vi "Split Single-line Message.vi"(2 "single-line text":string) -> (6 "operator":string, 7 "state":string, 9 "args":string, 10 "source/target":string)   [LabVIEW 2017, in "CSM Shared.lvlib"]
uses:
  CSM Shared.lvlib
  <vilib>/regexp/Match Regular Expression.xnode
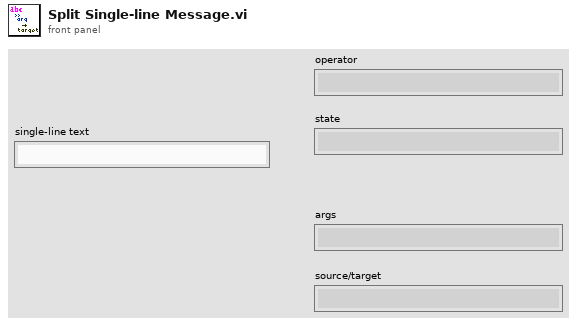
[diagram p1: front panel]
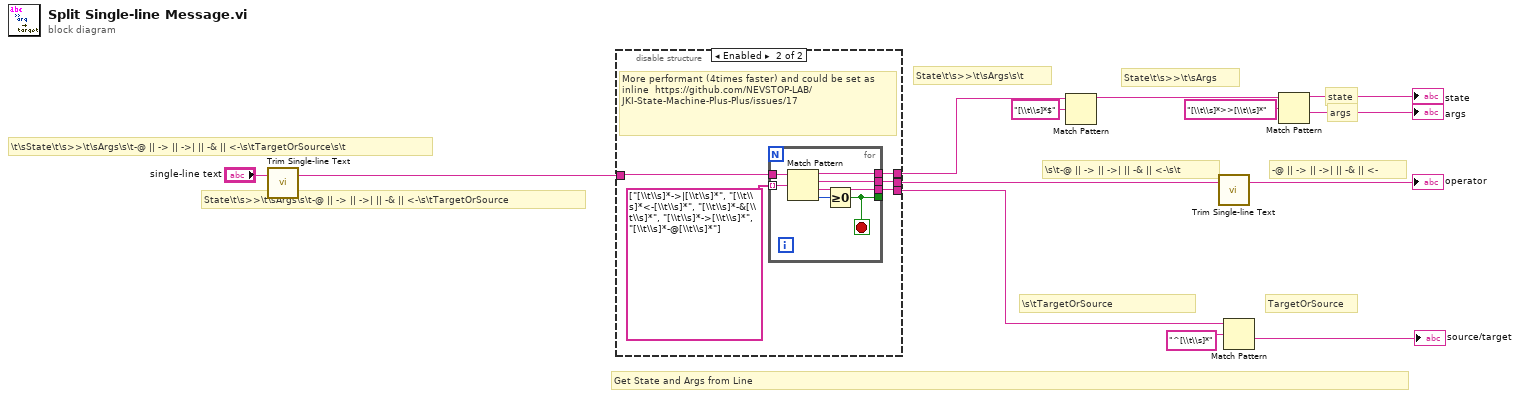
[diagram p0: block diagram]
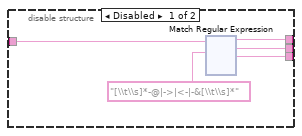
[diagram p2: hidden frame]
diagram:
  # "TargetOrSource"
  # "\\t\\sState\\t\\s>>\\t\\sArgs\\s\\t-@ || -> || ->| || -& || <-\\s\\tTargetOrSource\\s\\t"
  # "-@ || -> || ->| || -& || <-"
  # "\\s\\t-@ || -> || ->| || -& || <-\\s\\t"
  # "State\\t\\s>>\\t\\sArgs"
  # "State\\t\\s>>\\t\\sArgs\\s\\t"
  # "Get State and Args from Line"
  # "State\\t\\s>>\\t\\sArgs\\s\\t-@ || -> || ->| || -& || <-\\s\\tTargetOrSource"
  # "\\s\\tTargetOrSource"
  # "args"
  # "state"
  n1 = call "Trim Single-line Text.vi"("single-line text"="single-line text") -> ("trimed text"=w1:string)  [unwired: 2 in]
  n2 = disable-structure shown="Enabled" {
    disable-tunnel: [w17 w135] -> w11
    disable-tunnel: [w16 w134] -> w5
    disable-tunnel: [w15 w133] -> w7
    disable-tunnel: w1 -> [w14 w137]
    frame Disabled {
      n3 = xnode "Match Regular Expression"("input string"=w14, "regular expression"="[\\t\\s]*-@|->|<-|-&[\\t\\s]*") -> ("before match"=w17:string, "whole match"=w16:string, "after match"=w15:string)  [unwired: 4 in, 2 out]
    }
    frame Enabled {
      # "More performant (4times faster) and could be set as inline  https://github.com/NEVSTOP-LAB/JKI-State-Machine-Plus-Plus/issues/17"
      n4 = for {
        tunnel: w137 -> [w144]
        tunnel: string[] ["[\\t\\s]*->|[\\t\\s]*", "[\\t\\s]*<-[\\t\\s]*", "[\\t\\s]*-&[\\t\\s]*", "[\\t\\s]*->[\\t\\s]*", "[\\t\\s]*-@[\\t\\s]*"] -> [w143] mode=indexing
        tunnel: [w141] -> _
        tunnel: [w140] -> w135
        tunnel: [w139] -> w134
        tunnel: [w138] -> w133
        stop <- w141 stop-if-true
        n5 = Match Pattern(string=w144, regular expression=w143) -> (before substring=w140:string, match substring=w139:string, after substring=w138:string, offset past match=w142:i32)  [unwired: 1 in]
        n6 = Greater Or Equal To 0?(x=w142) -> (x >= 0?=w141:bool)
      }
    }
  }
  n7 = Match Pattern(string=w11, regular expression="[\\t\\s]*$") -> (before substring=w10:string)  [unwired: 1 in, 3 out]
  n8 = call "Trim Single-line Text.vi"("single-line text"=w5) -> ("trimed text"=→"operator":string)  [unwired: 2 in]
  n9 = Match Pattern(string=w7, regular expression="^[\\t\\s]*") -> (after substring=→"source/target":string)  [unwired: 1 in, 3 out]
  n10 = Match Pattern(string=w10, regular expression="[\\t\\s]*>>[\\t\\s]*") -> (before substring=→"state":string, after substring=→"args":string)  [unwired: 1 in, 2 out]
